vi "ServiceStatusSignals.Compile.vi"(8 "error in (no error)":errorcluster, 10 "Settings":T1[](array[typedef]) {"Signal.Cmd.Refs"."Signal Refs" format="%.0x"; "Signal.Cmd.Info"."Signals"."Byte Order" items=["Little Endian", "Big Endian"]; "Signal.Cmd.Info"."Signals"."Data Type" items=["Signed", "Unsigned", "IEEE Float"]; "Settings.Refs"."Signal Refs" format="%.0x"; "Signal.Resp.Refs"."Signal Refs" format="%.0x"; "Signal.Resp.Info"."Signals"."Byte Order" items=["Little Endian", "Big Endian"]; "Signal.Resp.Info"."Signals"."Data Type" items=["Signed", "Unsigned", "IEEE Float"]; "Trigger.Refs"."Signal Refs" format="%.0x"; "Status.Refs"."Signal Refs" format="%.0x"}) -> (0 "error out":errorcluster, 2 "Refs":T7 {"VS Refs" format="%.0x"}, 3 "Status Lookup":variant)   [LabVIEW 2019, in "Diagnostics Addon System Explorer.lvlib"]
uses:
  Diagnostics Addon System Explorer.lvlib
  <vilib>/NI VeriStand/Custom Device API/Custom Device Item Ref.ctl
  Types/Service.Export.ctl
  Types/Frame.Ref.ctl
  Shared/Types/Type.ctl
  Shared/Types/Frame.Compile.ctl
  Shared/Types/Signal.ctl
  Shared/Types/ServiceChannels.LookupType.ctl
  Shared/SubVIs/Constants.vi
  <vilib>/NI VeriStand/Custom Device API/Custom Device API.lvlib
  Shared/Diagnostics Addon Shared.lvlib
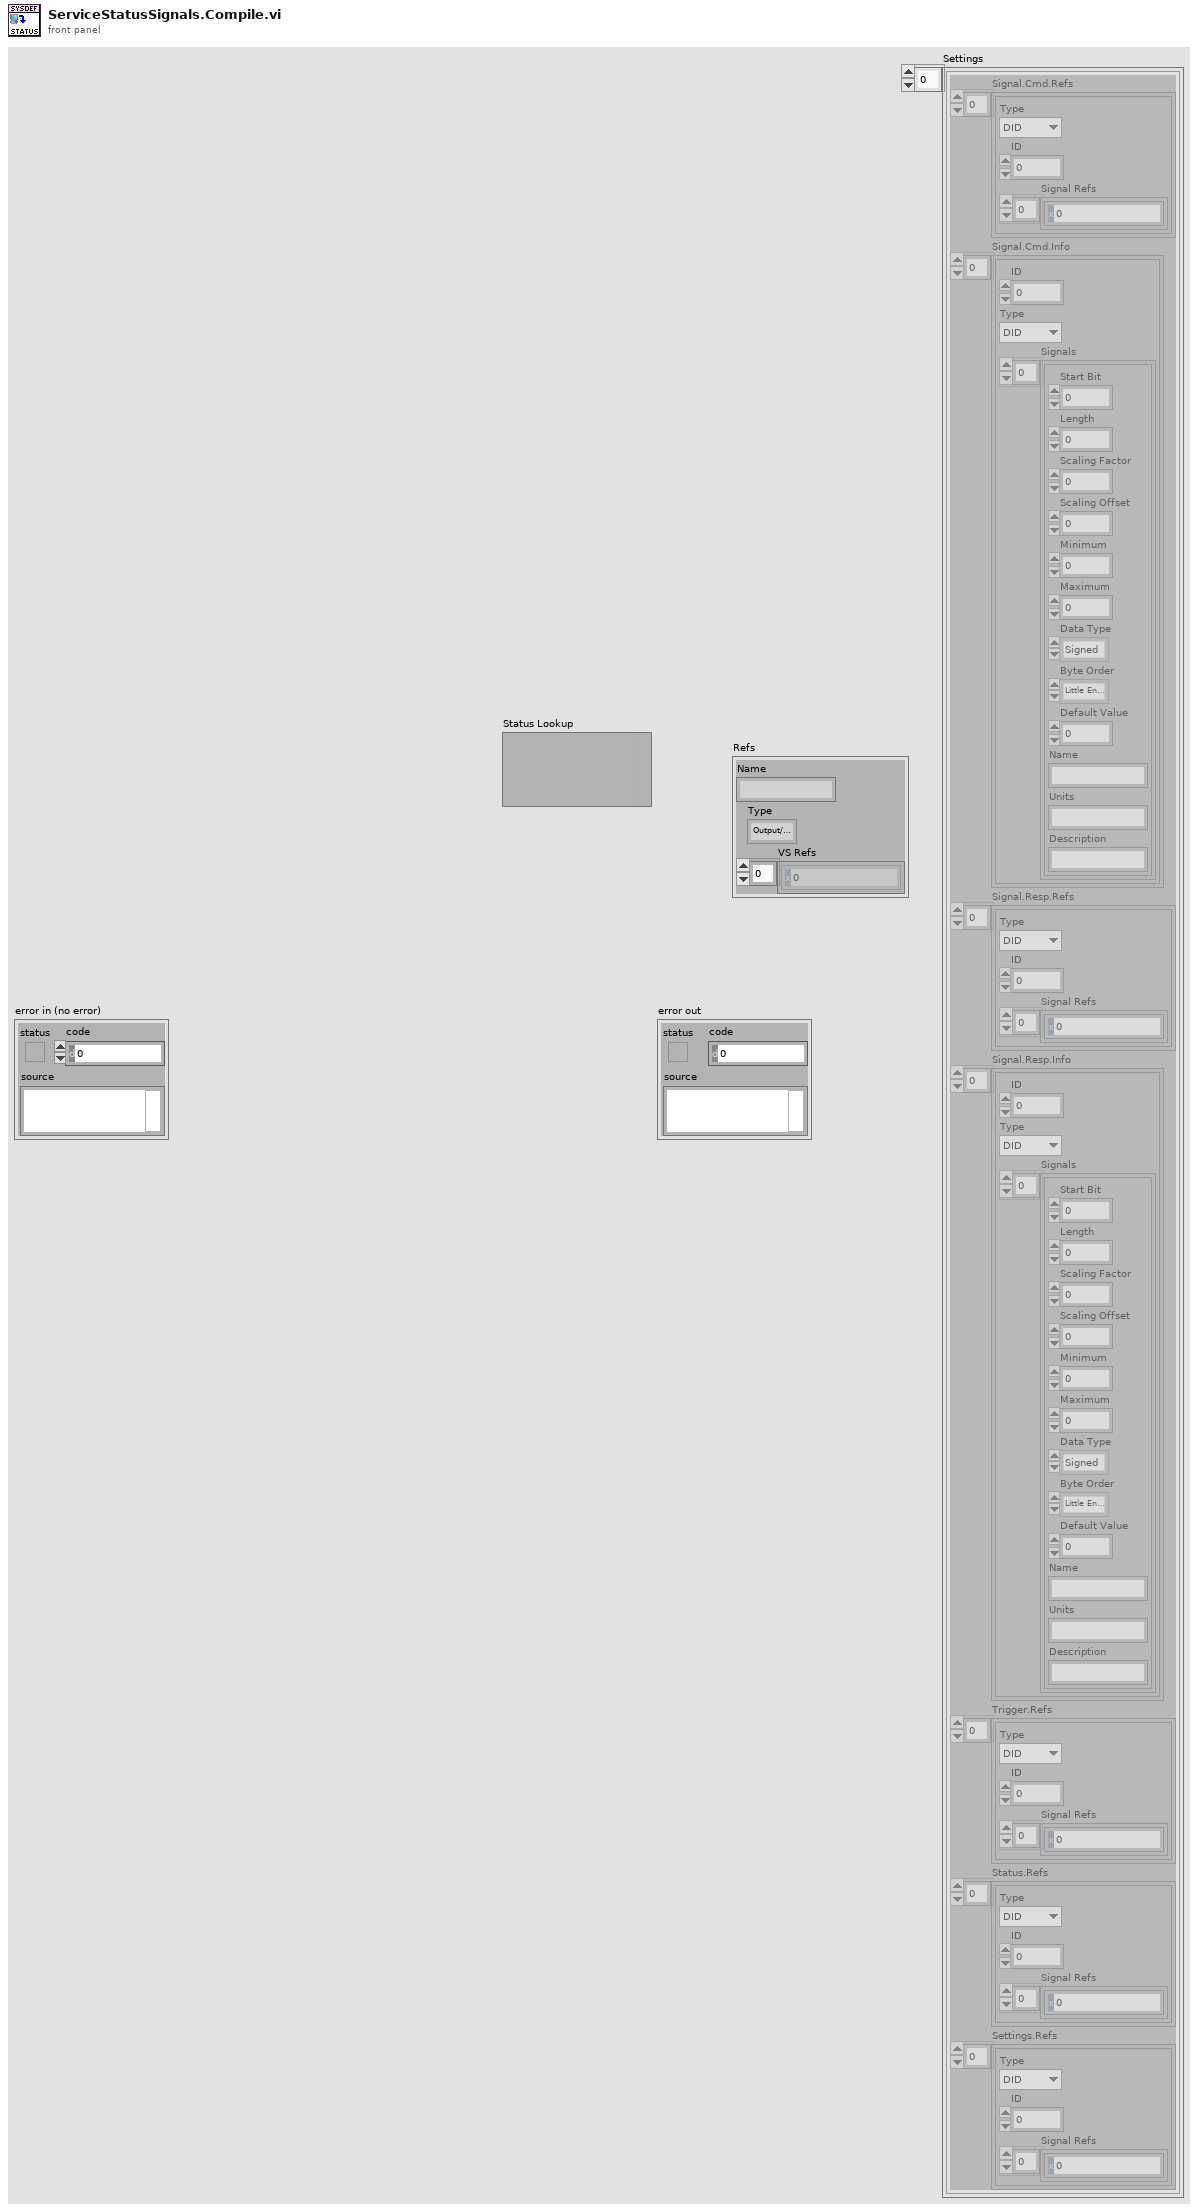
[diagram p1: front panel]
types:
  T1 = typedef "Diagnostics Addon System Explorer.lvlib/Service.Export.ctl" = cluster{"Signal.Cmd.Refs":T2[], "Signal.Cmd.Info":T5[], "Signal.Resp.Refs":T2[], "Signal.Resp.Info":T5[], "Trigger.Refs":T2[], "Status.Refs":T2[], "Settings.Refs":T2[]}
  T2 = typedef "Diagnostics Addon System Explorer.lvlib/Frame.Ref.ctl" = cluster{"Type":T3, "ID":u32, "Signal Refs":T4[]}
  T3 = typedef "Diagnostics Addon Shared.lvlib/Type.ctl" = enum16{"DID", "CDID", "PID", "CPID", "Read Memory", "Write Memory", "DTC Control", "IO Cmd", "IO Resp", "Routine Start Cmd", "Routine Start Resp", "Routine Request Cmd", "Routine Request Resp", "Routine Stop Cmd", "Routine Stop Resp", "UserDefined Cmd", "UserDefined Rsp"}
  T4 = typedef "Custom Device API.lvlib/Custom Device Item Ref.ctl" = u64
  T5 = typedef "Diagnostics Addon Shared.lvlib/Frame.Compile.ctl" = cluster{"ID":u32, "Type":T3, "Signals":T6[]}
  T6 = typedef "Diagnostics Addon Shared.lvlib/Signal.ctl" = cluster{"Start Bit":u32, "Length":u32, "Scaling Factor":dbl, "Scaling Offset":dbl, "Minimum":dbl, "Maximum":dbl, "Data Type":u32, "Byte Order":u32, "Default Value":dbl, "Name":string, "Units":string, "Description":string}
  T7 = cluster{"Name":string, "Type":enum16{"Output/Write", "Input/Read", "Input/ReadWrite"}, "VS Refs":T4[]}
  T8 = enum16{"Output/Write", "Input/Read", "Input/ReadWrite"}
  T9 = typedef "Diagnostics Addon Shared.lvlib/ServiceChannels.LookupType.ctl" = cluster{"Offset":i32}
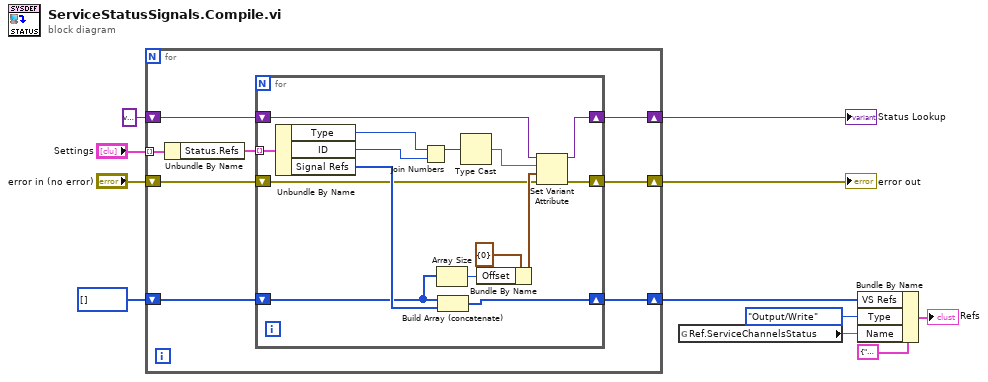
[diagram p0: block diagram]
diagram:
  n1 = for {
    shift-right: [w14] -> w3
    shift-left: "error in (no error)" -> [w19]
    shift-right: [w18] -> w10
    shift-left: variant ("Lookup In") -> [w16]
    shift-right: [w15] -> w4
    shift-left: T4[] [] -> [w17]
    tunnel: "Settings" -> [w13] mode=indexing
    n2 = Unbundle By Name(w13) -> ("Status.Refs"=w12:T2[])
    n3 = for {
      tunnel: w12 -> [w28] mode=indexing
      shift-right: [w29] -> w18
      shift-left: w16 -> [w33]
      shift-right: [w31] -> w14
      shift-left: w19 -> [w24]
      shift-right: [w27] -> w15
      shift-left: w17 -> [w25]
      n4 = Unbundle By Name(w28) -> ("Type"=w21:T3, "ID"=w23:u32, "Signal Refs"=w26:T4[])
      n5 = Join Numbers(hi=w21, lo=w23) -> ((hi.lo)=w22:u64)
      n6 = Array Size(array=w25) -> (size(s)=w32:i32)
      n7 = Build Array (concatenate)(w25, w26) -> (w27:T4[])
      n8 = Type Cast(x=w22) -> (*(type *) &x=w30:string)  [unwired: 1 in]
      n9 = Bundle By Name(cluster=T9 {"Offset"=0}, "Offset"=w32) -> (w34:T9)
      n10 = Set Variant Attribute(Variant=w33, name=w30, value=w34, error in=w24) -> (Variant out=w29:variant, error out=w31:errorcluster)  [unwired: 1 out]
    }
  }
  "error out" <- w3
  "Status Lookup" <- w10
  n11 = global read "Constants.vi" "Ref.ServiceChannelsStatus"() -> (w7:string)
  n12 = Bundle By Name(cluster=T7 {"Name"="", "Type"=enum."Output/Write", "VS Refs"=[]} ("Group"), "VS Refs"=w4, "Type"=T8."Output/Write", "Name"=w7) -> (→"Refs":T7)
